vi "Configure_Voltage.vi"(6 "Measurement Type":T1(ring), 8 "error in (no error)":errorcluster, 9 "Resolution in Digits":T2(ring)=enum."5 1/2", 10 "Range":dbl=10.0 format="%.2f", 11 "KeysightDmm in":refnum<class "KeysightDmm.lvclass">) -> (0 "error out":errorcluster, 3 "KeysightDmm out":refnum<class "KeysightDmm.lvclass">)   [LabVIEW 2021, in "KeysightDmm.lvclass"]
uses:
  KeysightDmm.lvclass
  KeysightDmm.lvclass/KeysightDmm.ctl
  <instrlib>/Agilent 34401/Agilent 34401.lvlib
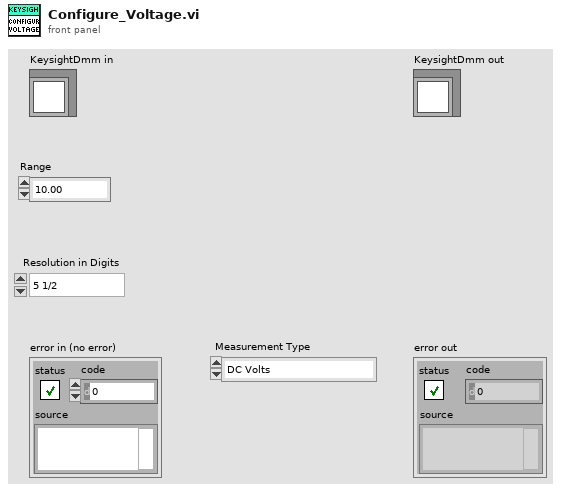
[diagram p1: front panel]
types:
  T1 = enum32{"DC Volts", "AC Volts", "DC Current", "AC Current", "2-wire Resistance", "4-wire Resistance", "Diode", "Frequency", "Period", "AC Volts DC Coupled", "Capacitance", "Inductance", "Temperature"}
  T2 = enum32{"3 1/2", "4 1/2", "5 1/2", "6 1/2", "7 1/2"}
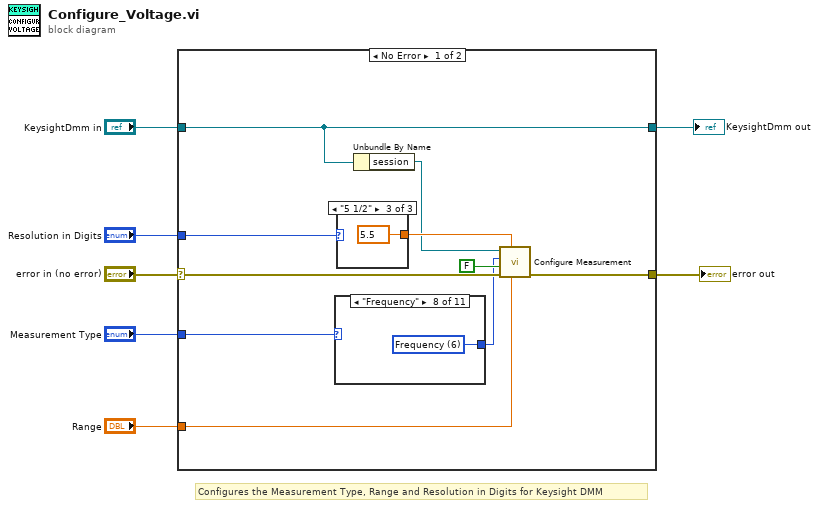
[diagram p0: block diagram]
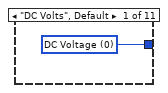
[diagram p2: hidden frame]
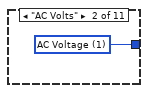
[diagram p3: hidden frame]
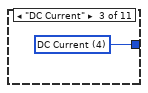
[diagram p4: hidden frame]
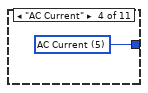
[diagram p5: hidden frame]
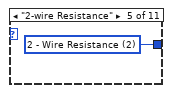
[diagram p6: hidden frame]
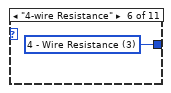
[diagram p7: hidden frame]
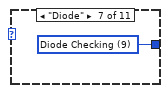
[diagram p8: hidden frame]
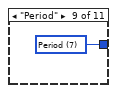
[diagram p9: hidden frame]
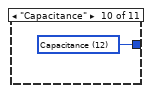
[diagram p10: hidden frame]
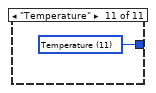
[diagram p11: hidden frame]
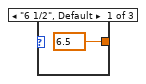
[diagram p12: hidden frame]
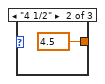
[diagram p13: hidden frame]
diagram:
  # "Configures the Measurement Type, Range and Resolution in Digits for Keysight DMM"
  n1 = case shown="No Error" "error in (no error)" {
    selector: "error in (no error)" -> [w17 w32]
    tunnel: [w16 w32] -> w6
    tunnel: "KeysightDmm in" -> [w12 w33]
    tunnel: [w12 w33] -> w4
    tunnel: "Range" -> [w10 _]
    tunnel: "Resolution in Digits" -> [w9 _]
    tunnel: "Measurement Type" -> [w8 _]
    frame No Error {
      n2 = case shown="\"Frequency\"" w8 {
        tunnel: [w18 w19 w20 w21 w22 w23 w24 w25 w26 w27 w28] -> w13
        frame "DC Volts", Default {
          w18 = u16 0 items=["DC Voltage", "AC Voltage", "2 - Wire Resistance", "4 - Wire Resistance", "DC Current", "AC Current", "Frequency", "Period", "Continuity", "Diode Checking", "VDC:VDC Ratio", "Temperature", "Capacitance"] ("Function (0: DC Voltage)")
        }
        frame "AC Volts" {
          w19 = u16 1 items=["DC Voltage", "AC Voltage", "2 - Wire Resistance", "4 - Wire Resistance", "DC Current", "AC Current", "Frequency", "Period", "Continuity", "Diode Checking", "VDC:VDC Ratio", "Temperature", "Capacitance"] ("Function (0: DC Voltage)")
        }
        frame "DC Current" {
          w20 = u16 4 items=["DC Voltage", "AC Voltage", "2 - Wire Resistance", "4 - Wire Resistance", "DC Current", "AC Current", "Frequency", "Period", "Continuity", "Diode Checking", "VDC:VDC Ratio", "Temperature", "Capacitance"] ("Function (0: DC Voltage)")
        }
        frame "AC Current" {
          w21 = u16 5 items=["DC Voltage", "AC Voltage", "2 - Wire Resistance", "4 - Wire Resistance", "DC Current", "AC Current", "Frequency", "Period", "Continuity", "Diode Checking", "VDC:VDC Ratio", "Temperature", "Capacitance"] ("Function (0: DC Voltage)")
        }
        frame "2-wire Resistance" {
          w22 = u16 2 items=["DC Voltage", "AC Voltage", "2 - Wire Resistance", "4 - Wire Resistance", "DC Current", "AC Current", "Frequency", "Period", "Continuity", "Diode Checking", "VDC:VDC Ratio", "Temperature", "Capacitance"] ("Function (0: DC Voltage)")
        }
        frame "4-wire Resistance" {
          w23 = u16 3 items=["DC Voltage", "AC Voltage", "2 - Wire Resistance", "4 - Wire Resistance", "DC Current", "AC Current", "Frequency", "Period", "Continuity", "Diode Checking", "VDC:VDC Ratio", "Temperature", "Capacitance"] ("Function (0: DC Voltage)")
        }
        frame "Diode" {
          w24 = u16 9 items=["DC Voltage", "AC Voltage", "2 - Wire Resistance", "4 - Wire Resistance", "DC Current", "AC Current", "Frequency", "Period", "Continuity", "Diode Checking", "VDC:VDC Ratio", "Temperature", "Capacitance"] ("Function (0: DC Voltage)")
        }
        frame "Frequency" {
          w25 = u16 6 items=["DC Voltage", "AC Voltage", "2 - Wire Resistance", "4 - Wire Resistance", "DC Current", "AC Current", "Frequency", "Period", "Continuity", "Diode Checking", "VDC:VDC Ratio", "Temperature", "Capacitance"] ("Function (0: DC Voltage)")
        }
        frame "Period" {
          w26 = u16 7 items=["DC Voltage", "AC Voltage", "2 - Wire Resistance", "4 - Wire Resistance", "DC Current", "AC Current", "Frequency", "Period", "Continuity", "Diode Checking", "VDC:VDC Ratio", "Temperature", "Capacitance"] ("Function (0: DC Voltage)")
        }
        frame "Capacitance" {
          w27 = u16 12 items=["DC Voltage", "AC Voltage", "2 - Wire Resistance", "4 - Wire Resistance", "DC Current", "AC Current", "Frequency", "Period", "Continuity", "Diode Checking", "VDC:VDC Ratio", "Temperature", "Capacitance"] ("Function (0: DC Voltage)")
        }
        frame "Temperature" {
          w28 = u16 11 items=["DC Voltage", "AC Voltage", "2 - Wire Resistance", "4 - Wire Resistance", "DC Current", "AC Current", "Frequency", "Period", "Continuity", "Diode Checking", "VDC:VDC Ratio", "Temperature", "Capacitance"] ("Function (0: DC Voltage)")
        }
      }
      n3 = case shown="\"5 1/2\"" w9 {
        tunnel: [w29 w30 w31] -> w15
        frame "6 1/2", Default {
          w29 = 6.5 items=["4.5"=4.5, "5.5"=5.5, "6.5"=6.5] ("Manual Resolution (5.5 Digits)")
        }
        frame "4 1/2" {
          w30 = 4.5 items=["4.5"=4.5, "5.5"=5.5, "6.5"=6.5] ("Manual Resolution (5.5 Digits)")
        }
        frame "5 1/2" {
          w31 = 5.5 items=["4.5"=4.5, "5.5"=5.5, "6.5"=6.5] ("Manual Resolution (5.5 Digits)")
        }
      }
      n4 = Unbundle By Name(w12) -> ("session"=w11:refnum<visa-resource-name>)
      n5 = call <instrlib>:"Configure Measurement.vi"("Manual Range (1.00)"=w10, "Manual Resolution (5.5 Digits)"=w15, "error in (no error)"=w17, "Enable Auto Range (T: Enable)"=FALSE, "Function (0: DC Voltage)"=w13, "VISA resource name"=w11) -> ("error out"=w16:errorcluster)  [unwired: 4 in, 1 out]
    }
    frame Error {
    }
  }
  "error out" <- w6
  "KeysightDmm out" <- w4
